vi "Get Application Log.vi"(6 "clear after (true)?":bool=TRUE, 8 "error in (no error)":errorcluster, 11 "JMP application":refnum<k7>) -> (0 "error out":errorcluster, 2 "JMP log":string, 3 "JMP application out":refnum<k7>)   [LabVIEW 2019, in "JMP Automation.lvlib"]
doc: "Returns the current contents of the Log window as a String. The Log Window can be floating or docked. If the log is hidden, an empty string is returned.\n\nclear after (true)? : if true the log is cleard after retrival"
uses:
  <instrlib>/LV_JMP_bridge/JMP Automation.lvlib
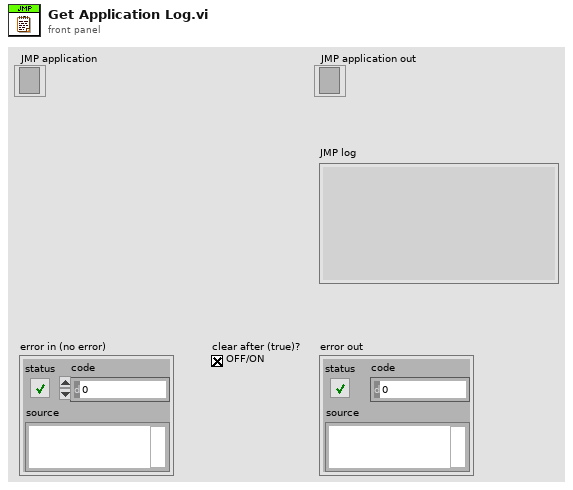
[diagram p1: front panel]
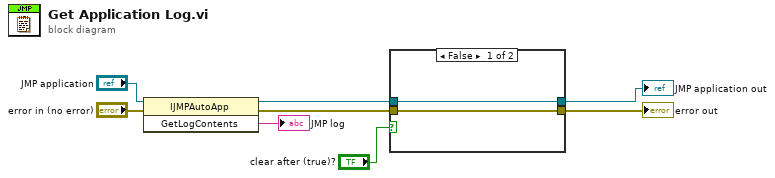
[diagram p0: block diagram]
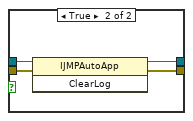
[diagram p2: hidden frame]
diagram:
  n1 = invoke class="IJMPAutoApp" method="GetLogContents"(reference="JMP application", error in="error in (no error)") -> (reference out=w4:refnum<k7>, error out=w3:errorcluster, "GetLogContents"=→"JMP log":string)  [unwired: 1 in]
  n2 = case shown="False" "clear after (true)?" {
    tunnel: w4 -> [w10 w14]
    tunnel: w3 -> [w9 w13]
    tunnel: [w10 w12] -> w2
    tunnel: [w9 w11] -> w1
    frame False {
    }
    frame True {
      n3 = invoke class="IJMPAutoApp" method="ClearLog"(reference=w14, error in=w13) -> (reference out=w12:refnum<k7>, error out=w11:errorcluster)  [unwired: 1 in, 1 out]
    }
  }
  "error out" <- w1
  "JMP application out" <- w2
